vi "UTILITY 1D String to 1D DBL.vi"(11 "Save Data":string[](array[string])) -> (3 "DBL":dbl[](array[numeric]))   [LabVIEW 2019]
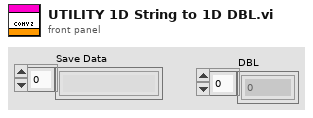
[diagram p1: front panel]
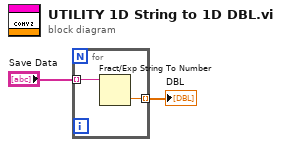
[diagram p0: block diagram]
diagram:
  n1 = for {
    tunnel: "Save Data" -> [w4] mode=indexing
    tunnel: [w3] -> w1 mode=indexing
    n2 = Fract/Exp String To Number(string=w4) -> (number=w3:dbl)  [unwired: 3 in, 1 out]
  }
  "DBL" <- w1
